vi "test - remove multiline Key.vi"(8 "error in (no error)":errorcluster, 11 "TestCase in":refnum<class "labview-config-library.lvclass">) -> (0 "error out":errorcluster, 3 "TestCase out":refnum<class "labview-config-library.lvclass">)   [LabVIEW 2017, in "labview-config-library.lvclass"]
uses:
  labview-config-library.lvclass
  <vilib>/addons/_JKI Toolkits/VI Tester/TestCase.llb/TestCase.lvclass
  INI-Static-Variable-Support/LabVIEW-Config/LabVIEW-Config.lvclass
  INI-Static-Variable-Support/LabVIEW-Config/Read Key (String).vi
  <userlib>/_NEVSTOP/Communicable State Machine(CSM)/Communicable State Machine.lvlib
  C:/Program Files (x86)/National Instruments/LabVIEW 2017/vi.lib/addons/_JKI Toolkits/VI Tester/TestCase.llb/TestCase.lvclass
panel:
  in  "Tab Control":enum32{"Page 1", "Page 2", "Page 3"}(tab)
  out "Value":string
  out "text":string
  out "Key Names":string[](array[string])
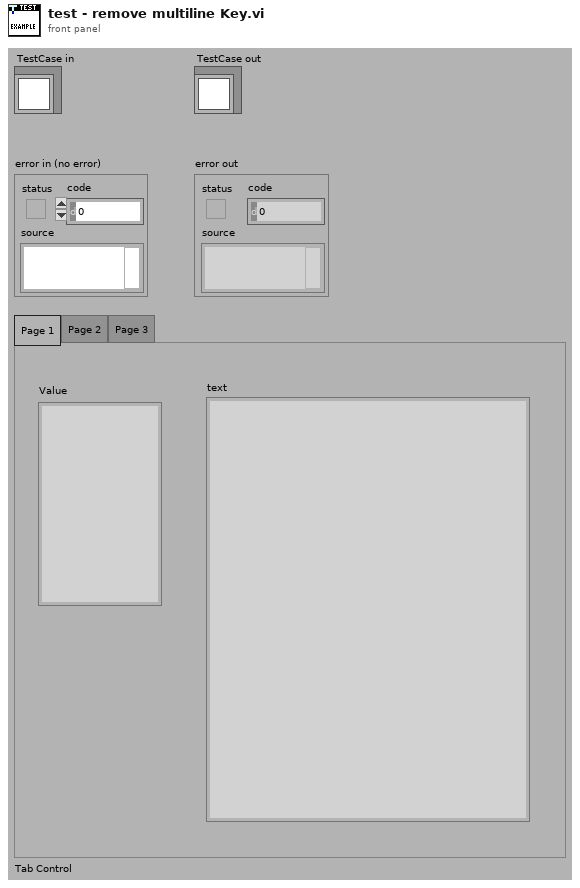
[diagram p1: front panel]
types:
  T1 = typedef "LabVIEW-Config.lvlib/LabVIEW-Config.lvclass/Config.ctl" = cluster{"Path":path, "Lines":string[], "Tokens":T2[], "Modified?":bool, "Cache":cluster{"Valid?":bool, "Key Information":T3[]}}
  T2 = typedef "LabVIEW-Config.lvlib/LabVIEW-Config.lvclass/LineToken.ctl" = enum8{"comment", "section", "key", "more"}
  T3 = typedef "LabVIEW-Config.lvlib/LabVIEW-Config.lvclass/KeyInfo.ctl" = cluster{"Key Indexes":cluster{"Indexes":i32[]}[], "Session Found?":bool, "Key found?":bool, "Session Index":i32}
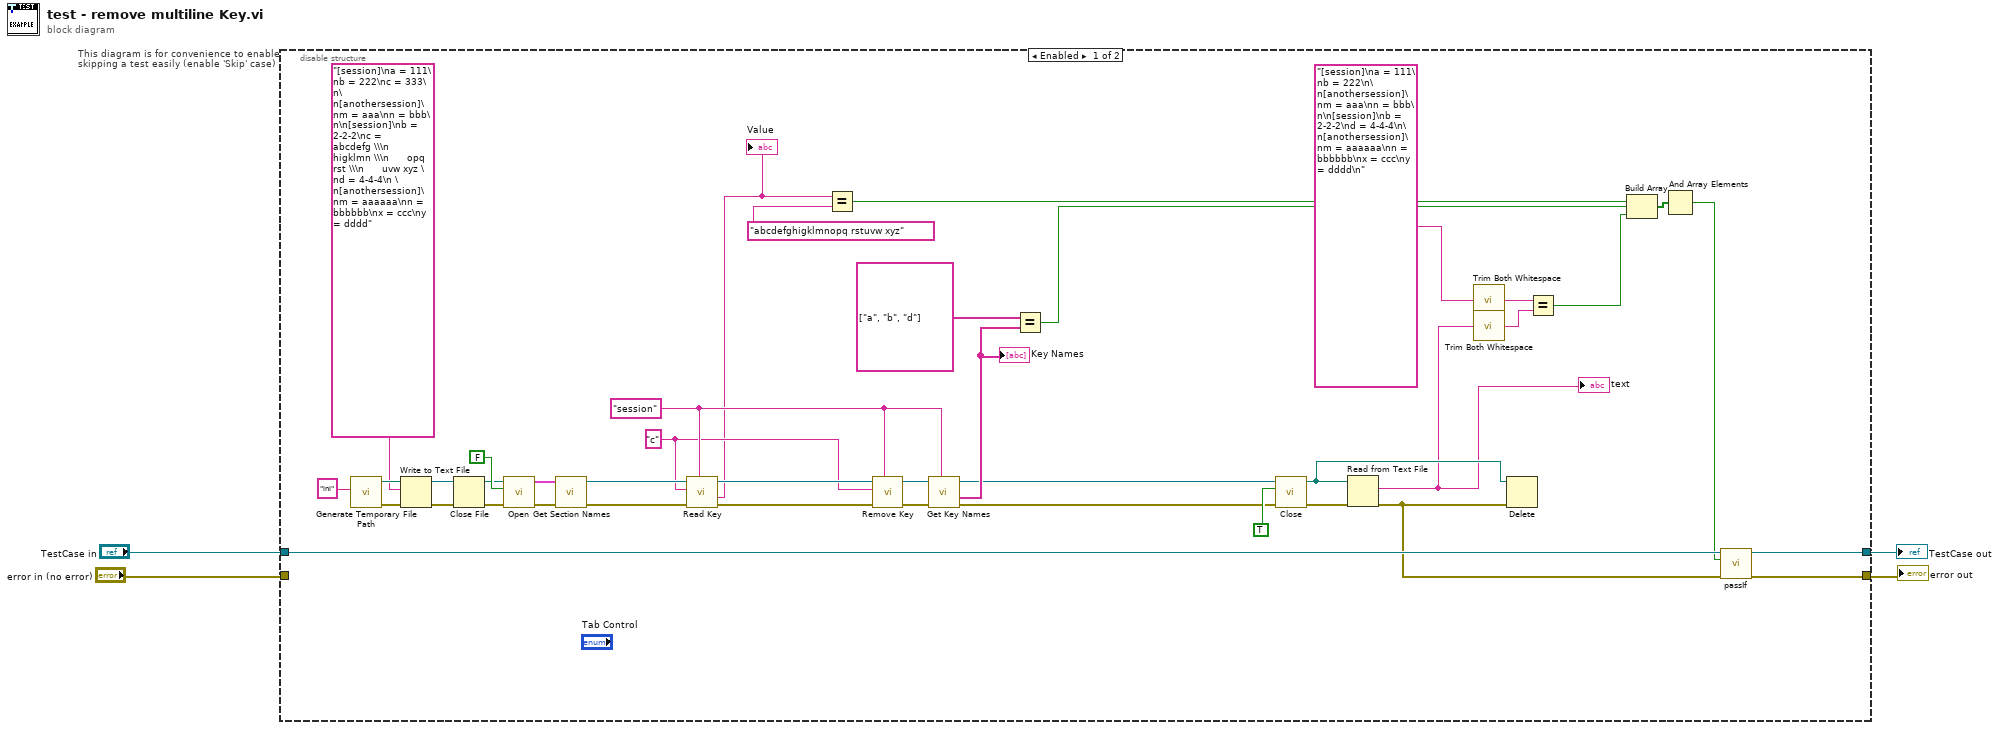
[diagram p0: block diagram]
diagram:
  n1 = disable-structure "This diagram is for convenience to enable skipping a test easily (enable 'Skip' case)" shown="Enabled" {
    disable-tunnel: "TestCase in" -> [w45 w49]
    disable-tunnel: [w44 w47] -> w1
    disable-tunnel: [w43 w48] -> w3
    disable-tunnel: "error in (no error)" -> [_ w46]
    frame Enabled {
      w13 = "c"
      w14 = "session" ("Section Name")
      # "Create temporary ini file"
      n2 = call <vilib>:"Generate Temporary File Path.vi"("Temporary File Extension (tmp)"="ini") -> ("error out"=w40:errorcluster, "Unique Temporary File Path"=w37:path)  [unwired: 9 in]
      n3 = Write to Text File(file (use dialog)=w37, text="[session]\na = 111\nb = 222\nc = 333\n\n[anothersession]\nm = aaa\nn = bbb\n\n[session]\nb = 2-2-2\nc = abcdefg \\\n      higklmn \\\n      opq rst \\\n      uvw xyz \nd = 4-4-4\n \n[anothersession]\nm = aaaaaa\nn = bbbbbb\nx = ccc\ny = dddd", error in=w40) -> (refnum out=w36:refnum<file>, error out=w38:errorcluster)  [unwired: 1 in, 1 out]
      n4 = Close File(refnum=w36, error in=w38) -> (path=w33:path, error out=w34:errorcluster)
      n5 = call "Open.vi"("error in (no error)"=w34, "Create if not exists? (T)"=FALSE, "Path"=w33) -> ("error out"=w31:errorcluster, "Config"=w32:T1)  [unwired: 5 in, 2 out]
      n6 = call "Get Section Names.vi"("error in (no error)"=w31, "Config in"=w32) -> ("error out"=w16:errorcluster, "Config out"=w30:refnum<class "LabVIEW-Config.lvclass">)  [unwired: 7 in, 1 out]
      n7 = call-poly "Read Key.vi"("Section Name"=w14, "error in (no error)"=w16, "Key Name"=w13, "Config in"=w30) -> ("error out"=w15:errorcluster, "Value"=w12:string, "Config out"=w17:refnum<class "LabVIEW-Config.lvclass">)  [unwired: 4 in, 1 out]
      "Value" <- w12
      n8 = Equal?(x=w12, y="abcdefghigklmnopq rstuvw xyz") -> (x = y?=w10:bool)
      n9 = call "Remove Key.vi"("Section Name"=w14, "error in (no error)"=w15, "Key Name"=w13, "Config in"=w17) -> ("error out"=w26:errorcluster, "Config out"=w27:refnum<class "LabVIEW-Config.lvclass">)  [unwired: 5 in, 1 out]
      n10 = call "Get Key Names.vi"("Section Name"=w14, "error in (no error)"=w26, "Config in"=w27) -> ("error out"=w21:errorcluster, "Key Names"=w24:string[], "Config out"=w22:refnum<class "LabVIEW-Config.lvclass">)  [unwired: 5 in, 1 out]
      "Key Names" <- w24
      n11 = Equal?(x=string[] ["a", "b", "d"] ("Key Names"), y=w24) -> (x = y?=w23:bool)
      n12 = call "Close.vi"("error in (no error)"=w21, "Write if modified? (T)"=TRUE, "Config"=w22) -> ("error out"=w19:errorcluster, "Path"=w20:path)  [unwired: 7 in]
      n13 = Read from Text File(file (use dialog)=w20, error in=w19) -> (text=w8:string, error out=w18:errorcluster)  [unwired: 2 in, 2 out]
      "text" <- w8
      n14 = call <userlib>:"Trim Both Whitespace.vi"("string"="[session]\na = 111\nb = 222\n\n[anothersession]\nm = aaa\nn = bbb\n\n[session]\nb = 2-2-2\nd = 4-4-4\n\n[anothersession]\nm = aaaaaa\nn = bbbbbb\nx = ccc\ny = dddd\n") -> ("trimmed string"=w5:string)  [unwired: 1 in]
      n15 = call <userlib>:"Trim Both Whitespace.vi"("string"=w8) -> ("trimmed string"=w6:string)  [unwired: 1 in]
      n16 = Delete(path (use dialog)=w20, error in=w18) -> ()  [unwired: 3 in, 3 out]
      n17 = Equal?(x=w5, y=w6) -> (x = y?=w7:bool)
      n18 = Build Array(w10, w23, w7) -> (w29:bool[])
      n19 = And Array Elements(Boolean array=w29) -> (logical AND=w28:bool)
      n20 = call-dynamic "passIf.vi"("error in (no error)"=w18, "pass"=w28, "TestCase in"=w45) -> ("error out"=w43:errorcluster, "TestCase out"=w44:refnum<class "labview-config-library.lvclass">)  [unwired: 7 in]
    }
    frame Disabled {
      # "skip test result while test is under development"
      n21 = call <vilib>:"skip.vi"("error in (no error)"=w46, "TestCase in"=w49) -> ("error out"=w48:errorcluster, "TestCase out"=w47:refnum<class "labview-config-library.lvclass">)  [unwired: 8 in]
    }
  }
  "error out" <- w3
  "TestCase out" <- w1
